vi "Convert Subnet Mask to Dotted Decimal.vi"(11 "Mask CIDR":u8) -> (2 "Mask":u32 format="%.0x", 3 "Mask":string)   [LabVIEW 2021, in "Networking_CIF_U.lvlib"]
uses:
  Networking_CIF_U.lvlib
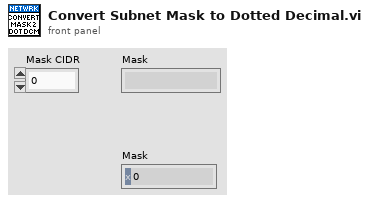
[diagram p1: front panel]
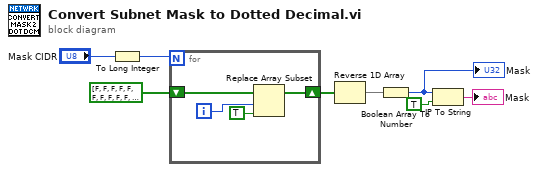
[diagram p0: block diagram]
diagram:
  n1 = To Long Integer(number="Mask CIDR") -> (32bit integer=w7:i32)
  n2 = for {
    N: w7 -> [_]
    shift-right: [w9] -> w5
    shift-left: bool[] [FALSE, FALSE, FALSE, FALSE, FALSE, FALSE, FALSE, FALSE, FALSE, FALSE, FALSE, FALSE, FALSE, FALSE, FALSE, FALSE, FALSE, FALSE, FALSE, FALSE, FALSE, FALSE, FALSE, FALSE, FALSE, FALSE, FALSE, FALSE, FALSE, FALSE, FALSE, FALSE] -> [w12]
    i -> [w11]
    n3 = Replace Array Subset(array=w12, new element=TRUE ("new element/subarray"), index=w11) -> (w9:bool[])
  }
  n4 = Reverse 1D Array(array=w5) -> (reversed array=w4:bool[])
  n5 = Boolean Array To Number(Boolean array=w4) -> (number=w3:u32)
  "Mask" <- w3
  n6 = IP To String(1:TRUE ("dot notation? (F)"), 2:w3) -> (0:→"Mask":string)
